vi "Invalidate All Attributes.vi"(8 "error in (no error)":errorcluster, 11 "CS++Scope":refnum<class "CS++Scope.lvclass">) -> (0 "error out":errorcluster, 3 "CS++Scope out":refnum<class "CS++Scope.lvclass">)   [LabVIEW 2016, in "CS++Scope.lvlib" / "CS++Scope.lvclass"]
doc: "This VI invalidates the cached values of all properties for the session."
uses:
  CS++Scope.lvclass
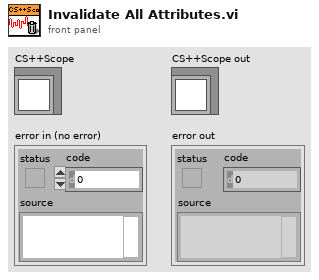
[diagram p1: front panel]
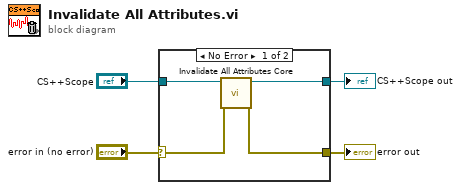
[diagram p0: block diagram]
diagram:
  n1 = case shown="No Error" "error in (no error)" {
    selector: "error in (no error)" -> [w6 w10]
    tunnel: [w5 w10] -> w3
    tunnel: [w7 w9] -> w2
    tunnel: "CS++Scope" -> [w8 w9]
    frame No Error {
      n2 = call-dynamic "Invalidate All Attributes Core.vi"("error in (no error)"=w6, "CS++Scope"=w8) -> ("error out"=w5:errorcluster, "CS++Scope out"=w7:refnum<class "CS++Scope.lvclass">)  [unwired: 8 in]
    }
    frame Error {
    }
  }
  "error out" <- w3
  "CS++Scope out" <- w2
